vi "string_concat_example.vi"() -> ()   [LabVIEW 2018]
uses:
  C:/Users/booko/Desktop/ENABLE/UpDownCounter/bin/Debug/netstandard2.0/UpDownCounter.dll
  UpDownCounter/bin/Debug/netstandard2.0/UpDownCounter.dll
panel:
  out "concatenateStrings":string
  in  "y":string
  in  "x":string
  in  "error in (no error)":errorcluster
  out "error out":errorcluster
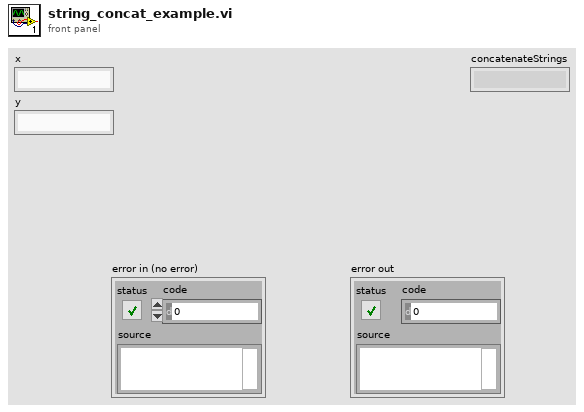
[diagram p1: front panel]
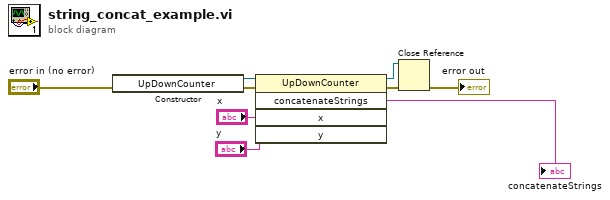
[diagram p0: block diagram]
diagram:
  n1 = constructor class="UpDownCounter"(error in="error in (no error)") -> (reference out=w9:refnum<k24>, error out=w7:errorcluster)  [unwired: 2 in, 1 out]
  n2 = invoke class="UpDownCounter" method="concatenateStrings"(reference=w9, error in=w7, "x"="x", "y"="y") -> (reference out=w8:refnum<k24>, error out=w6:errorcluster, "concatenateStrings"=→"concatenateStrings":string)  [unwired: 1 in, 2 out]
  n3 = Close Reference(reference=w8, error in (no error)=w6) -> (error out=→"error out":errorcluster)
